vi "PhotronPDCMessageLoop.vi"(8 "Error In":errorcluster, 11 "CommunicationRefs":T1) -> (0 "Error Out":errorcluster)   [LabVIEW 2015]
uses:
  TypeDefs/CommunicationRefs.ctl
  TypeDefs/MessageCluster.ctl
  TypeDefs/PDCSettings.ctl
  TypeDefs/PDCRecordStatus.ctl
  TypeDefs/PDCAllStates.ctl
  TypeDefs/PDCDisplay.ctl
  TypeDefs/PDCSaveSettings.ctl
  TypeDefs/PDCLists.ctl
  TypeDefs/PDCSetup.ctl
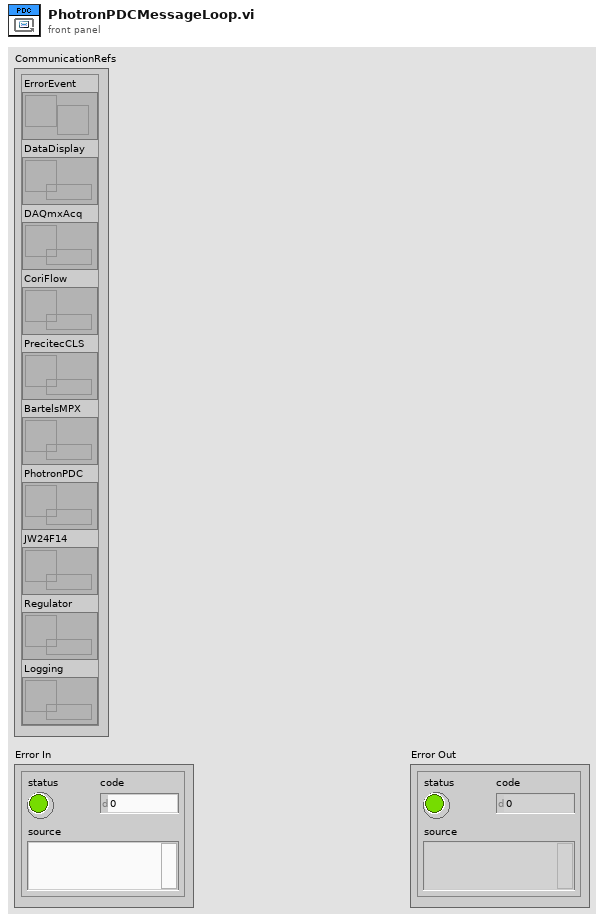
[diagram p1: front panel]
types:
  T1 = typedef "CommunicationRefs.ctl" = cluster{"ErrorEvent":refnum<user-event>, "DataDisplay":refnum<queue>, "DAQmxAcq":refnum<queue>, "CoriFlow":refnum<queue>, "PrecitecCLS":refnum<queue>, "BartelsMPX":refnum<queue>, "PhotronPDC":refnum<queue>, "JW24F14":refnum<queue>, "Regulator":refnum<queue>, "Logging":refnum<queue>}
  T2 = typedef "PDCRecordStatus.ctl" = enum16{"Live", "Endless", "Recording"}
  T3 = typedef "PDCSaveSettings.ctl" = cluster{"Save Folder":path, "File Name":string, "Data Type":enum16{"BMP", "AVI", "MRAW"}}
  T4 = cluster{"PDC Save Settings":T3, "SaveStatus":refnum<vi>}
  T5 = typedef "PDCAllStates.ctl" = cluster{"DeviceNo":u32, "ChildNo":u32, "ColorType":enum16{"MONO", "COLOR"}, "BitDepth":i8, "Resolution":cluster{"Width":u32, "Height":u32}, "RecordRate":u32, "ShutterSpeed":u32, "TriggerMode":u32, "Display":T6, "PDCRecordStatus":T2, "PlayFrames":bool, "Start Frame":i32, "Current Frame":i32, "End Frame":i32, "RefImage8bit":u8[], "RefImage16bit":u16[], "Auto Trigger":bool, "PDCSettings":T7}
  T6 = typedef "PDCDisplay.ctl" = enum16{"Live", "Memory", "LiveStop"}
  T7 = typedef "PDCSettings.ctl" = cluster{"Interface":enum16{"Gigabit-Ethernet", "IEEE1394a", "Photron Optical", "PCI/PCI Express"}, "AutoSearch":bool, "IP - AutoSearch":u32[], "IP - Direct":u32[], "Simulate":bool}
  T8 = typedef "PDCLists.ctl" = cluster{"ResolutionList":string[], "RecordRateList":string[], "ShutterSpeedList":string[], "TriggerModeList":string[]}
  T9 = typedef "PDCSetup.ctl" = cluster{"Color Type":enum16{"MONO", "COLOR"}, "Bit Depth":i8, "Resolution":u16, "Record Rate":u16, "Shutter Speed":u16, "Trigger Mode":u16, "Display":T6, "Auto Trigger":bool}
  T10 = cluster{"Start":i32, "End":i32, "Trigger":i32, "TwoStageLowToHigh":i32, "TwoStageHighToLow":i32, "TwoStageTiming":u32, "Event":i32[], "EventCount":u32, "RecordedFrames":u32}
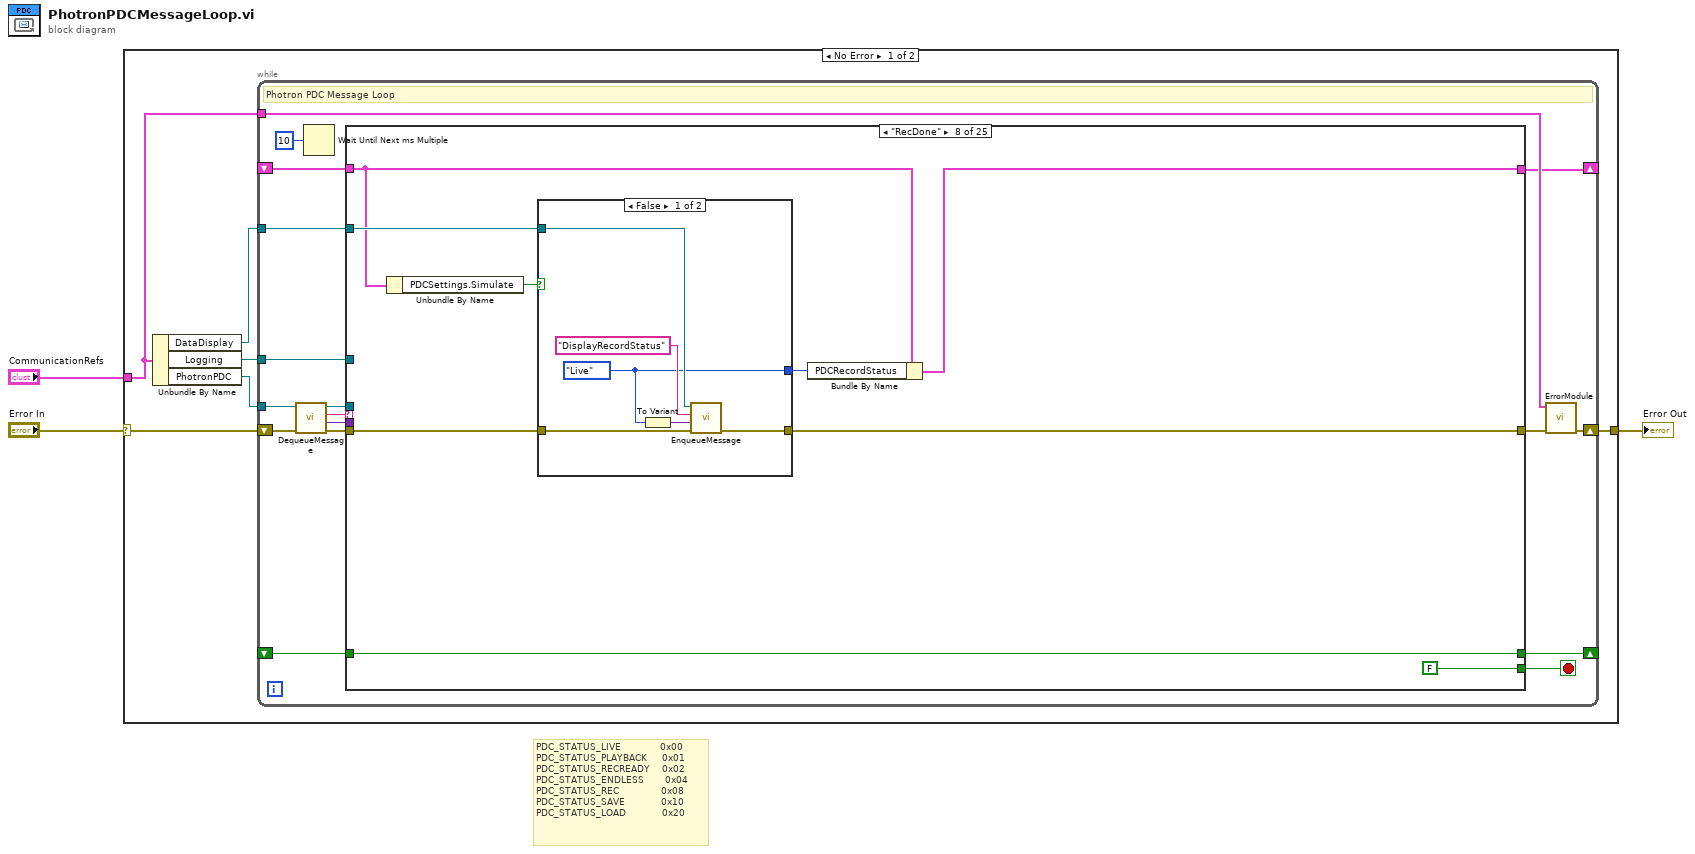
[diagram p0: block diagram]
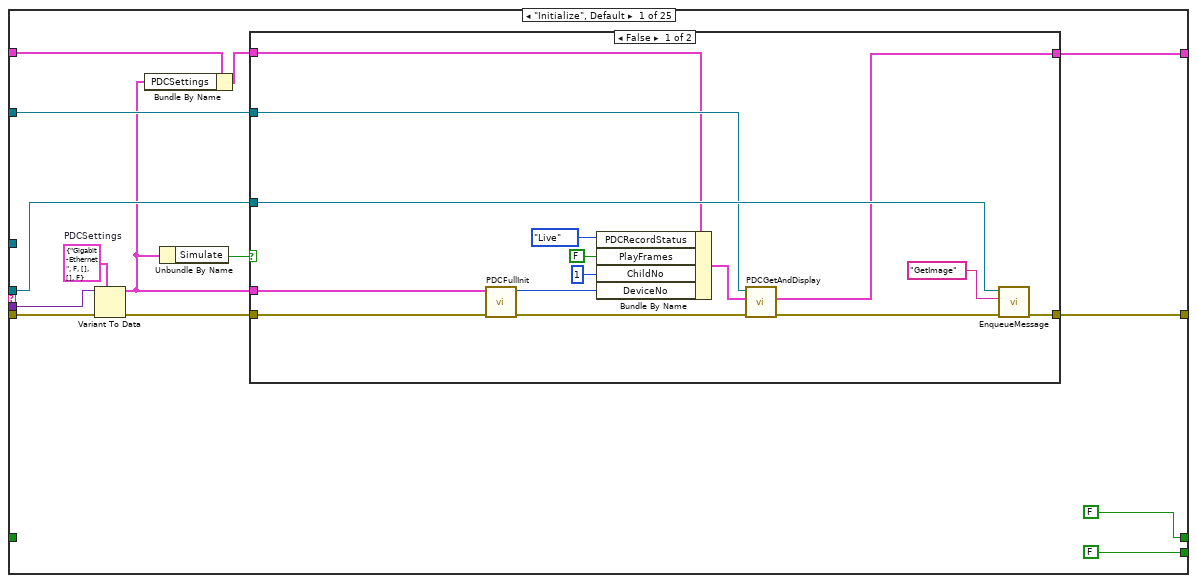
[diagram p2: hidden frame]
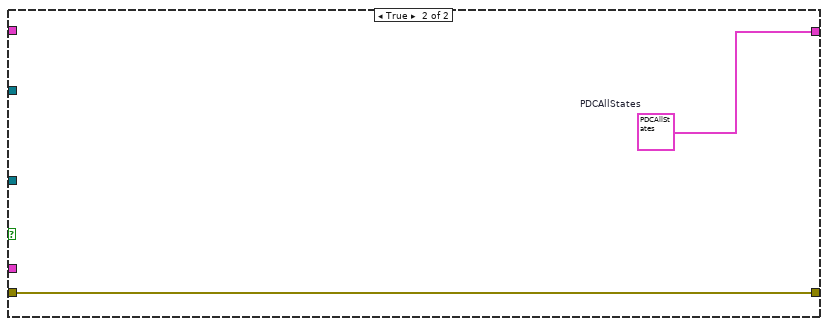
[diagram p3: hidden frame]
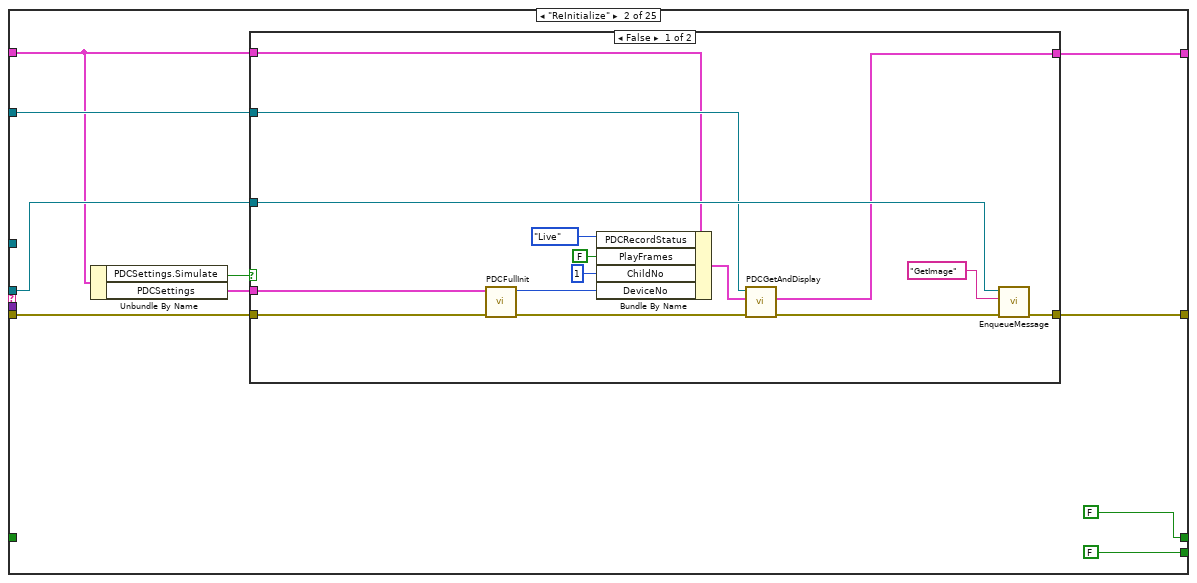
[diagram p4: hidden frame]
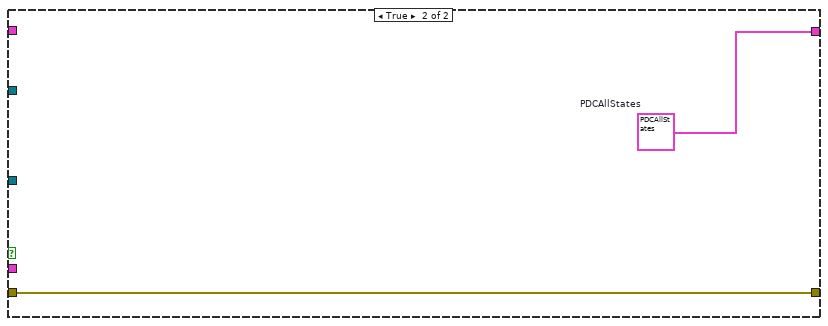
[diagram p5: hidden frame]
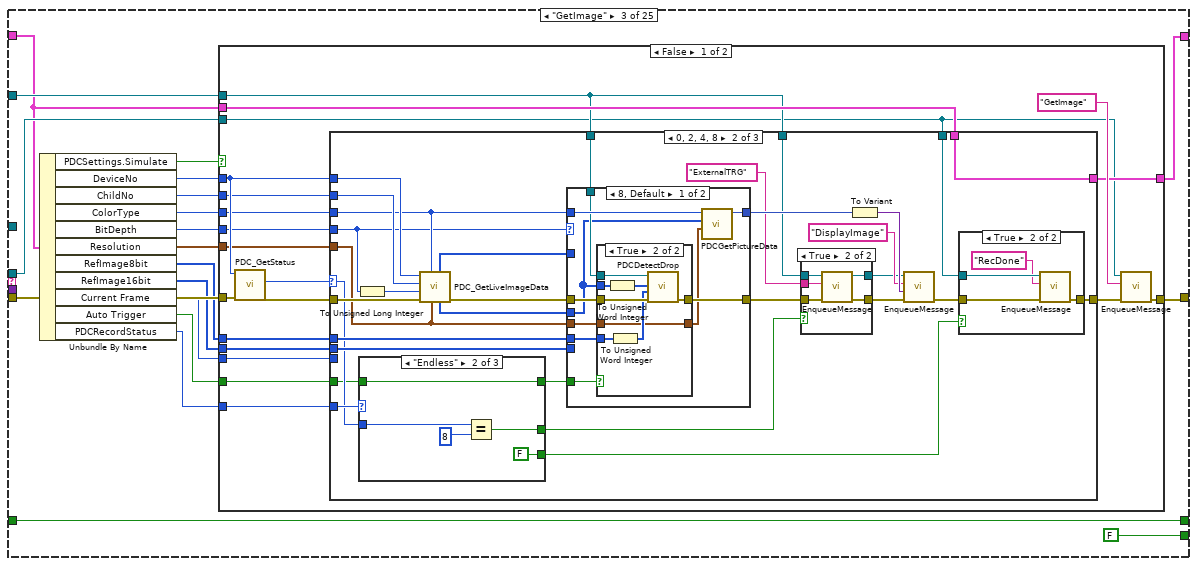
[diagram p6: hidden frame]
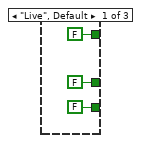
[diagram p9: hidden frame]
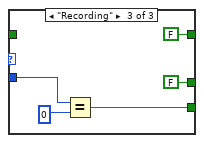
[diagram p10: hidden frame]
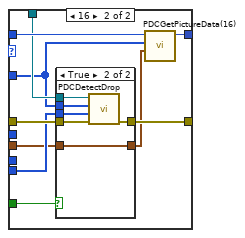
[diagram p13: hidden frame]
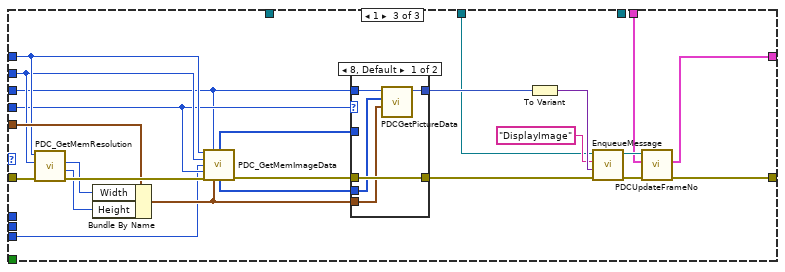
[diagram p15: hidden frame]
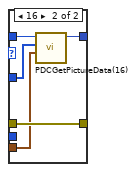
[diagram p16: hidden frame]
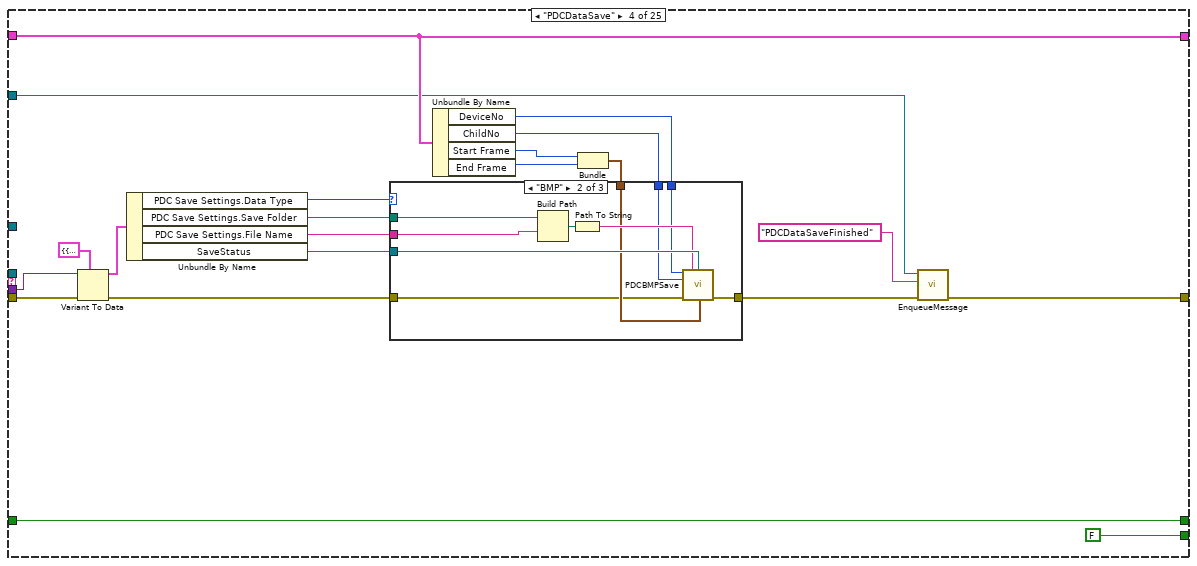
[diagram p18: hidden frame]
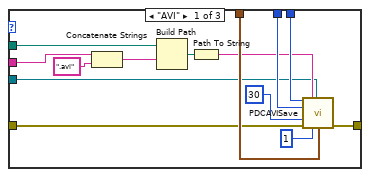
[diagram p19: hidden frame]
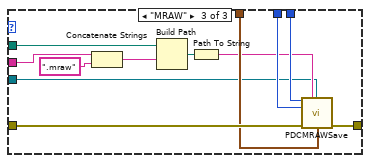
[diagram p20: hidden frame]
diagram:
  # "PDC_STATUS_LIVE\t\t\t\t\t\t       0x00\nPDC_STATUS_PLAYBACK\t\t\t\t\t0x01\nPDC_STATUS_RECREADY\t\t\t\t0x02\nPDC_STATUS_ENDLESS\t\t\t\t\t  0x04\nPDC_STATUS_REC\t\t\t\t\t\t        0x08\nPDC_STATUS_SAVE\t\t\t\t\t       0x10\nPDC_STATUS_LOAD\t\t\t\t\t\t      0x20"
  n1 = case shown="No Error" "Error In" {
    selector: "Error In" -> [w8 w753]
    tunnel: [w7 w753] -> w2
    tunnel: "CommunicationRefs" -> [w6 _]
    frame No Error {
      n2 = Unbundle By Name(w6) -> ("DataDisplay"=w5:refnum<queue>, "Logging"=w4:refnum<queue>, "PhotronPDC"=w9:refnum<queue>)
      n3 = while {
        tunnel: w9 -> [w26]
        tunnel: w6 -> [w18]
        shift-right: [w20] -> w7
        shift-left: w8 -> [w25]
        tunnel: w5 -> [w16]
        tunnel: w4 -> [w15]
        shift-right: [w14] -> _
        shift-left: _ -> [w13]
        shift-right: [w12] -> _
        shift-left: _ -> [w11]
        stop <- w17 stop-if-true
        # "Photron PDC Message Loop"
        n4 = call "DequeueMessage.vi"("error in (no error)"=w25, "MessageQueue"=w26) -> ("error out"=w21:errorcluster, "MessageData"=w22:variant, "Message"=w23:string, "dupMessageQueue"=w24:refnum<queue>)  [unwired: 6 in]
        n5 = Wait Until Next ms Multiple(millisecond multiple=u32 10) -> ()  [unwired: 1 out]
        n6 = case shown="\"RecDone\"" w23 {
          tunnel: w24 -> [w33 w63 w93 _ w313 w357 _ _ _ _ _ _ _ _ _ _ _ _ _ _ _ _ _ _ w742]
          tunnel: w22 -> [w30 _ _ w267 w321 _ _ _ w428 w437 w448 w457 w466 w480 w525 w577 w602 w627 w654 w679 w704 _ _ _ _]
          tunnel: w21 -> [w37 w58 w101 w268 w323 w364 w395 w415 w436 w445 w454 w463 w472 w482 w527 w579 w604 w629 w656 w681 w706 w721 w728 w733 w741]
          tunnel: [w38 w65 w95 w259 w324 w358 w396 w416 w431 w440 w451 w460 w469 w484 w529 w581 w606 w631 w658 w683 w708 w721 w728 w732 w747] -> w19
          tunnel: [FALSE FALSE FALSE FALSE FALSE FALSE FALSE FALSE FALSE FALSE FALSE FALSE FALSE FALSE FALSE FALSE FALSE FALSE FALSE FALSE FALSE FALSE FALSE TRUE FALSE] -> w17
          tunnel: w16 -> [w34 w64 w94 w257 w317 _ w393 w414 _ _ _ _ _ w475 w519 w572 w597 w623 w649 w674 w699 _ _ _ _]
          tunnel: w15 -> [_ _ _ _ _ _ _ _ _ _ _ _ _ _ _ _ _ _ _ _ _ _ _ _ _]
          tunnel: [FALSE FALSE w91 w275 w327 w354 w399 w419 w430 w439 w450 w459 w468 w486 w531 w583 w608 w633 w660 w685 w710 TRUE FALSE FALSE w743] -> w14
          tunnel: w13 -> [_ _ w91 w275 w327 w354 w399 w419 w430 w439 w450 w459 w468 w486 w531 w583 w608 w633 w660 w685 w710 _ _ _ w743]
          tunnel: [w31 w61 w92 w274 w315 w355 w391 w412 w432 w441 w452 w461 w470 w477 w521 w574 w599 w625 w651 w676 w701 w722 w725 w731 w746] -> w12
          tunnel: w11 -> [w29 w60 w87 w274 w316 w356 w392 w413 w434 w443 w453 w462 w471 w474 w518 w570 w595 w620 w647 w672 w697 w722 w725 w731 w746]
          frame "Initialize", Default {
            w35 = T7 {"Interface"=enum."Gigabit-Ethernet", "AutoSearch"=FALSE, "IP - AutoSearch"=[], "IP - Direct"=[], "Simulate"=FALSE}  # PDCSettings
            n7 = Variant To Data(error in=w37, type=w35, Variant=w30) -> (data=w28:T7, error out=w36:errorcluster)
            n8 = Bundle By Name(cluster=w29, "PDCSettings"=w28) -> (w27:T5)
            n9 = Unbundle By Name(w28) -> ("Simulate"=w32:bool)
            n10 = case shown="False" w32 {
              tunnel: [w52 w57] -> w38
              tunnel: w36 -> [w54 w57]
              tunnel: w34 -> [w48 _]
              tunnel: w33 -> [w53 _]
              tunnel: [w50 w56] -> w31
              tunnel: w28 -> [w47 _]
              tunnel: w27 -> [w43 _]
              frame False {
                n11 = call "PDCFullInit.vi"("error in (no error)"=w54, "PDCSettings"=w47) -> ("error out"=w49:errorcluster, "DeviceNo"=w46:u32)  [unwired: 8 in]
                n12 = Bundle By Name(cluster=w43, "PDCRecordStatus"=PDCRecordStatus."Live", "PlayFrames"=FALSE, "ChildNo"=u32 1, "DeviceNo"=w46) -> (w44:T5)
                n13 = call "PDCGetAndDisplay.vi"("error in (no error)"=w49, "PDCAllStates in"=w44, "DataDisplayQueue"=w48) -> ("error out"=w55:errorcluster, "PDCAllStates out"=w50:T5)  [unwired: 7 in]
                n14 = call "EnqueueMessage.vi"("error in (no error)"=w55, "Message"="GetImage", "MessageQueue"=w53) -> ("error out"=w52:errorcluster)  [unwired: 7 in, 1 out]
              }
              frame True {
                w56 = T5 {"DeviceNo"=0, "ChildNo"=1, "ColorType"=enum."MONO", "BitDepth"=0, "Resolution"={"Width"=0, "Height"=0}, "RecordRate"=0, "ShutterSpeed"=0, "TriggerMode"=0, "Display"=enum."LiveStop", "PDCRecordStatus"=enum."Live", "PlayFrames"=FALSE, "Start Frame"=0, "Current Frame"=0, "End Frame"=0, "RefImage8bit"=[], "RefImage16bit"=[], "Auto Trigger"=FALSE, "PDCSettings"={"Interface"=enum."Gigabit-Ethernet", "AutoSearch"=FALSE, "IP - AutoSearch"=[], "IP - Direct"=[], "Simulate"=FALSE}}  # PDCAllStates
              }
            }
          }
          frame "ReInitialize" {
            n15 = Unbundle By Name(w60) -> ("PDCSettings.Simulate"=w62:bool, "PDCSettings"=w59:T7)
            n16 = case shown="False" w62 {
              tunnel: [w79 w84] -> w65
              tunnel: w58 -> [w81 w84]
              tunnel: w64 -> [w75 _]
              tunnel: w63 -> [w80 _]
              tunnel: [w77 w83] -> w61
              tunnel: w59 -> [w74 _]
              tunnel: w60 -> [w70 _]
              frame False {
                n17 = call "PDCFullInit.vi"("error in (no error)"=w81, "PDCSettings"=w74) -> ("error out"=w76:errorcluster, "DeviceNo"=w73:u32)  [unwired: 8 in]
                n18 = Bundle By Name(cluster=w70, "PDCRecordStatus"=PDCRecordStatus."Live", "PlayFrames"=FALSE, "ChildNo"=u32 1, "DeviceNo"=w73) -> (w71:T5)
                n19 = call "PDCGetAndDisplay.vi"("error in (no error)"=w76, "PDCAllStates in"=w71, "DataDisplayQueue"=w75) -> ("error out"=w82:errorcluster, "PDCAllStates out"=w77:T5)  [unwired: 7 in]
                n20 = call "EnqueueMessage.vi"("error in (no error)"=w82, "Message"="GetImage", "MessageQueue"=w80) -> ("error out"=w79:errorcluster)  [unwired: 7 in, 1 out]
              }
              frame True {
                w83 = T5 {"DeviceNo"=0, "ChildNo"=1, "ColorType"=enum."MONO", "BitDepth"=0, "Resolution"={"Width"=0, "Height"=0}, "RecordRate"=0, "ShutterSpeed"=0, "TriggerMode"=0, "Display"=enum."LiveStop", "PDCRecordStatus"=enum."Live", "PlayFrames"=FALSE, "Start Frame"=0, "Current Frame"=0, "End Frame"=0, "RefImage8bit"=[], "RefImage16bit"=[], "Auto Trigger"=FALSE, "PDCSettings"={"Interface"=enum."Gigabit-Ethernet", "AutoSearch"=FALSE, "IP - AutoSearch"=[], "IP - Direct"=[], "Simulate"=FALSE}}  # PDCAllStates
              }
            }
          }
          frame "GetImage" {
            n21 = Unbundle By Name(w87) -> ("PDCSettings.Simulate"=w102:bool, "DeviceNo"=w100:u32, "ChildNo"=w99:u32, "ColorType"=w98:enum16{"MONO", "COLOR"}, "BitDepth"=w97:i8, "Resolution"=w96:cluster{"Width":u32, "Height":u32}, "RefImage8bit"=w88:u8[], "RefImage16bit"=w89:u16[], "Current Frame"=w90:i32, "Auto Trigger"=w85:bool, "PDCRecordStatus"=w86:T2)
            n22 = case shown="False" w102 {
              tunnel: w101 -> [w123 w255]
              tunnel: w100 -> [w122 _]
              tunnel: w99 -> [w121 _]
              tunnel: w98 -> [w118 _]
              tunnel: w97 -> [w119 _]
              tunnel: w96 -> [w116 _]
              tunnel: [w115 w255] -> w95
              tunnel: w94 -> [w107 _]
              tunnel: w93 -> [w104 _]
              tunnel: w87 -> [w112 w254]
              tunnel: [w111 w254] -> w92
              tunnel: w90 -> [w110 _]
              tunnel: w89 -> [w109 _]
              tunnel: w88 -> [w108 _]
              tunnel: w86 -> [w106 _]
              tunnel: w85 -> [w105 _]
              frame False {
                n23 = call "PDC_GetStatus.vi"("error in (no error)"=w123, "DeviceNo"=w122) -> ("error out"=w120:errorcluster, "Status"=w117:u32)  [unwired: 6 in, 2 out]
                n24 = case shown="0, 2, 4, 8" w117 {
                  selector: w117 -> [_ w133 _]
                  tunnel: w122 -> [_ w156 w238]
                  tunnel: w121 -> [_ w155 w237]
                  tunnel: w120 -> [w125 w154 w242]
                  tunnel: w119 -> [_ w147 w233]
                  tunnel: w118 -> [_ w148 w232]
                  tunnel: w116 -> [_ w151 w241]
                  tunnel: [w125 w128 w224] -> w113
                  tunnel: w107 -> [_ w142 w226]
                  tunnel: w112 -> [w124 w138 w222]
                  tunnel: [w124 w138 w221] -> w111
                  tunnel: w110 -> [_ _ w220]
                  tunnel: w109 -> [_ w136 _]
                  tunnel: w108 -> [_ w137 _]
                  tunnel: w107 -> [_ w135 _]
                  tunnel: w105 -> [_ w132 _]
                  tunnel: w106 -> [_ w134 _]
                  tunnel: w104 -> [_ w126 _]
                  frame Default {
                  }
                  frame 0, 2, 4, 8 {
                    n25 = To Unsigned Long Integer(number=w147) -> (unsigned 32bit integer=w153:u32)
                    n26 = case shown="\"Endless\"" w134 {
                      tunnel: w133 -> [_ w167 w171]
                      tunnel: w132 -> [_ w169 _]
                      tunnel: [FALSE ("Auto Trigger") w169 FALSE ("Auto Trigger")] -> w131
                      tunnel: [FALSE w166 FALSE] -> w130
                      tunnel: [FALSE FALSE w170] -> w127
                      frame "Live", Default {
                      }
                      frame "Endless" {
                        n27 = Equal?(x=w167, y=u32 8) -> (x = y?=w166:bool)
                      }
                      frame "Recording" {
                        n28 = Equal?(x=w171, y=u32 0) -> (x = y?=w170:bool)
                      }
                    }
                    n29 = call "PDC_GetLiveImageData.vi"("Resolution"=w151, "ColorType"=w148, "error in (no error)"=w154, "BitDepth"=w153, "ChildNo"=w155, "DeviceNo"=w156) -> ("error out"=w152:errorcluster, "Data(8Bit)"=w150:u8[], "Data(16Bit)"=w149:u16[])  [unwired: 1 in, 2 out]
                    n30 = case shown="8, Default" w147 {
                      tunnel: w148 -> [w191 w211]
                      tunnel: w151 -> [w183 w203]
                      tunnel: w150 -> [w185 _]
                      tunnel: w152 -> [w189 w209]
                      tunnel: [w188 w208] -> w140
                      tunnel: w149 -> [_ w205]
                      tunnel: [w190 w210] -> w144
                      tunnel: w137 -> [w186 _]
                      tunnel: w136 -> [_ w206]
                      tunnel: w135 -> [w187 w207]
                      tunnel: w131 -> [w184 w204]
                      frame 8, Default {
                        n31 = case shown="True" w184 {
                          tunnel: w189 -> [w192 w201]
                          tunnel: [w192 w200] -> w188
                          tunnel: w187 -> [_ w199]
                          tunnel: w186 -> [_ w198]
                          tunnel: w185 -> [_ w196]
                          tunnel: w183 -> [w193 w194]
                          tunnel: [w193 w194] -> w182
                          frame False {
                          }
                          frame True {
                            n32 = To Unsigned Word Integer(number=w196) -> (unsigned 16bit integer=w195:u16[])
                            n33 = To Unsigned Word Integer(number=w198) -> (unsigned 16bit integer=w197:u16[])
                            n34 = call "PDCDetectDrop.vi"("Error In"=w201, "RefImage"=w197, "CurrentImage"=w195, "DataDisplay"=w199) -> ("Error Out"=w200:errorcluster)  [unwired: 7 in]
                          }
                        }
                        n35 = call "PDCGetPictureData.vi"("Resolution"=w182, "Data(8Bit)"=w185, "ColorType"=w191) -> ("new picture"=w190:picture)  [unwired: 4 in]
                      }
                      frame 16 {
                        n36 = case shown="True" w204 {
                          tunnel: w209 -> [w212 w219]
                          tunnel: [w212 w218] -> w208
                          tunnel: w207 -> [_ w217]
                          tunnel: w206 -> [_ w216]
                          tunnel: w205 -> [_ w215]
                          tunnel: [w213 w214] -> w202
                          tunnel: w203 -> [w213 w214]
                          frame False {
                          }
                          frame True {
                            n37 = call "PDCDetectDrop.vi"("Error In"=w219, "RefImage"=w216, "CurrentImage"=w215, "DataDisplay"=w217) -> ("Error Out"=w218:errorcluster)  [unwired: 7 in]
                          }
                        }
                        n38 = call "PDCGetPictureData(16).vi"("Resolution"=w202, "Data(16Bit)"=w205, "ColorType"=w211) -> ("new picture"=w210:picture)  [unwired: 4 in]
                      }
                    }
                    n39 = case shown="True" w130 {
                      tunnel: [w176 w181] -> w143
                      tunnel: w142 -> [w175 w178]
                      tunnel: [w175 w177] -> w141
                      tunnel: w140 -> [w176 w180]
                      tunnel: "ExternalTRG" ("Message") -> [_ w179]
                      frame False {
                      }
                      frame True {
                        n40 = call "EnqueueMessage.vi"("error in (no error)"=w180, "Message"=w179, "MessageQueue"=w178) -> ("error out"=w181:errorcluster, "dupMessageQueue"=w177:refnum<queue>)  [unwired: 7 in]
                      }
                    }
                    n41 = To Variant(anything=w144) -> (Variant=w146:variant)
                    n42 = call "EnqueueMessage.vi"("error in (no error)"=w143, "MessageData"=w146, "Message"="DisplayImage", "MessageQueue"=w141) -> ("error out"=w129:errorcluster)  [unwired: 6 in, 1 out]
                    n43 = case shown="True" w127 {
                      tunnel: w126 -> [_ w161]
                      tunnel: w129 -> [w157 w160]
                      tunnel: [w157 w159] -> w128
                      frame False {
                      }
                      frame True {
                        n44 = call "EnqueueMessage.vi"("error in (no error)"=w160, "Message"="RecDone", "MessageQueue"=w161) -> ("error out"=w159:errorcluster)  [unwired: 7 in, 1 out]
                      }
                    }
                  }
                  frame 1 {
                    n45 = call "PDC_GetMemResolution.vi"("error in (no error)"=w242, "ChildNo"=w237, "DeviceNo"=w238) -> ("error out"=w243:errorcluster, "Height"=w240:u32, "Width"=w239:u32)  [unwired: 4 in, 2 out]
                    n46 = Bundle By Name(cluster=w241, "Width"=w239, "Height"=w240) -> (w235:cluster{"Width":u32, "Height":u32})
                    n47 = call "PDC_GetMemImageData.vi"("DeviceNo"=w238, "ColorType"=w232, "ChildNo"=w237, "FrameNo"=w220, "BitDepth"=w233, "error in (no error)"=w243, "Resolution"=w235) -> ("Data(16Bit)"=w231:u16[], "Data(8Bit)"=w234:u8[], "error out"=w236:errorcluster)  [unwired: 4 in, 2 out]
                    n48 = case shown="8, Default" w233 {
                      tunnel: w232 -> [w247 w252]
                      tunnel: w235 -> [w246 w251]
                      tunnel: w234 -> [w245 _]
                      tunnel: w236 -> [w248 w253]
                      tunnel: [w248 w253] -> w230
                      tunnel: w231 -> [_ w250]
                      tunnel: [w244 w249] -> w229
                      frame 8, Default {
                        n49 = call "PDCGetPictureData.vi"("Resolution"=w246, "Data(8Bit)"=w245, "ColorType"=w247) -> ("new picture"=w244:picture)  [unwired: 4 in]
                      }
                      frame 16 {
                        n50 = call "PDCGetPictureData(16).vi"("Resolution"=w251, "Data(16Bit)"=w250, "ColorType"=w252) -> ("new picture"=w249:picture)  [unwired: 4 in]
                      }
                    }
                    n51 = To Variant(anything=w229) -> (Variant=w228:variant)
                    n52 = call "EnqueueMessage.vi"("error in (no error)"=w230, "MessageData"=w228, "Message"="DisplayImage", "MessageQueue"=w226) -> ("error out"=w225:errorcluster, "dupMessageQueue"=w223:refnum<queue>)  [unwired: 6 in]
                    n53 = call "PDCUpdateFrameNo.vi"("Error In"=w225, "PDCAllStates in"=w222, "DataDisplayQueue"=w223) -> ("Error Out"=w224:errorcluster, "PDCAllStates out"=w221:T5)  [unwired: 7 in]
                  }
                }
                n54 = call "EnqueueMessage.vi"("error in (no error)"=w113, "Message"="GetImage", "MessageQueue"=w104) -> ("error out"=w115:errorcluster)  [unwired: 7 in, 1 out]
              }
              frame True {
              }
            }
          }
          frame "PDCDataSave" {
            n55 = Variant To Data(error in=w268, type=T4 {"PDC Save Settings"={"Save Folder"=path "", "File Name"="", "Data Type"=enum."AVI"}, "SaveStatus"=refnum} ("cluster"), Variant=w267) -> (data=w265:T4, error out=w264:errorcluster)
            n56 = Unbundle By Name(w265) -> ("PDC Save Settings.Data Type"=w260:enum16{"BMP", "AVI", "MRAW"}, "PDC Save Settings.Save Folder"=w262:path, "PDC Save Settings.File Name"=w261:string, "SaveStatus"=w263:refnum<vi>)
            n57 = Unbundle By Name(w274) -> ("DeviceNo"=w273:u32, "ChildNo"=w272:u32, "Start Frame"=w271:i32, "End Frame"=w270:i32)
            n58 = Bundle("Start Frame"=w271, "End Frame"=w270) -> (w269:cluster{"Start Frame":i32, "End Frame":i32})  [unwired: 1 in]
            n59 = case shown="\"BMP\"" w260 {
              tunnel: [w290 w294 w307] -> w258
              tunnel: w273 -> [w289 w296 w303]
              tunnel: w272 -> [w288 w295 w304]
              tunnel: w269 -> [w287 w293 w305]
              tunnel: w264 -> [w282 w292 w306]
              tunnel: w263 -> [w281 w298 w301]
              tunnel: w262 -> [w280 w299 w311]
              tunnel: w261 -> [w279 w291 w310]
              frame "AVI" {
                n60 = Concatenate Strings(w279, ".avi" ("string")) -> (w278:string)
                n61 = Build Path(base path=w280, name or relative path=w278) -> (appended path=w284:path)
                n62 = Path To String(path=w284) -> (string=w283:string)
                n63 = call "PDCAVISave.vi"("DeviceNo"=w289, "FileName"=w283, "Slide Refnum"=w281, "ChildNo"=w288, "Rate"=30, "error in (no error)"=w282, "ShowCompreddDlg"=u32 1, "File_Frame"=w287) -> ("error out"=w290:errorcluster)  [unwired: 7 in]
              }
              frame "BMP" {
                n64 = Build Path(base path=w299, name or relative path=w291) -> (appended path=w300:path)
                n65 = Path To String(path=w300) -> (string=w297:string)
                n66 = call "PDCBMPSave.vi"("DeviceNo"=w296, "FileName"=w297, "Slide Refnum"=w298, "ChildNo"=w295, "error in (no error)"=w292, "File_Frame"=w293) -> ("error out"=w294:errorcluster)  [unwired: 9 in]
              }
              frame "MRAW" {
                n67 = Concatenate Strings(w310, ".mraw" ("string")) -> (w309:string)
                n68 = Build Path(base path=w311, name or relative path=w309) -> (appended path=w312:path)
                n69 = Path To String(path=w312) -> (string=w302:string)
                n70 = call "PDCMRAWSave.vi"("DeviceNo"=w303, "FileName"=w302, "Slide Refnum"=w301, "ChildNo"=w304, "error in (no error)"=w306, "File_Frame"=w305) -> ("error out"=w307:errorcluster)  [unwired: 9 in]
              }
            }
            n71 = call "EnqueueMessage.vi"("error in (no error)"=w258, "Message"="PDCDataSaveFinished", "MessageQueue"=w257) -> ("error out"=w259:errorcluster)  [unwired: 7 in, 1 out]
          }
          frame "Record" {
            n72 = Unbundle By Name(w316) -> ("PDCSettings.Simulate"=w325:bool, "DeviceNo"=w318:u32)
            n73 = Variant To Data(error in=w323, type=PDCRecordStatus."Live" ("PDCRecordState"), Variant=w321) -> (data=w319:T2, error out=w322:errorcluster)
            n74 = case shown="False" w325 {
              tunnel: w322 -> [w335 w353]
              tunnel: [w333 w353] -> w324
              tunnel: w319 -> [w337 _]
              tunnel: w318 -> [w336 _]
              tunnel: w317 -> [w332 _]
              tunnel: [w329 PDCRecordStatus."Live" ("PDCRecordState")] -> w314
              tunnel: w313 -> [w328 _]
              frame False {
                n75 = case shown="\"Live\", Default" w337 {
                  tunnel: w336 -> [w339 w347 _]
                  tunnel: w335 -> [w340 w349 w351]
                  tunnel: [w344 w348 w351] -> w334
                  tunnel: [PDCRecordStatus."Endless" ("PDCRecordState") PDCRecordStatus."Recording" ("PDCRecordState") PDCRecordStatus."Recording" ("PDCRecordState")] -> w329
                  tunnel: w328 -> [w343 _ _]
                  frame "Live", Default {
                    n76 = call "PDC_SetEndless.vi"("error in (no error)"=w340, "DeviceNo"=w339) -> ("error out"=w338:errorcluster)  [unwired: 7 in, 2 out]
                    n77 = call "EnqueueMessage.vi"("Priority Message? (F)"=TRUE, "error in (no error)"=w338, "Message"="SetRefImage", "MessageQueue"=w343) -> ("error out"=w344:errorcluster)  [unwired: 6 in, 1 out]
                  }
                  frame "Endless" {
                    n78 = call "PDC_TriggerIn.vi"("error in (no error)"=w349, "DeviceNo"=w347) -> ("error out"=w348:errorcluster)  [unwired: 7 in, 2 out]
                  }
                  frame "Recording" {
                  }
                }
                n79 = To Variant(anything=w329) -> (Variant=w330:variant)
                n80 = call "EnqueueMessage.vi"("error in (no error)"=w334, "MessageData"=w330, "Message"="DisplayRecordStatus", "MessageQueue"=w332) -> ("error out"=w333:errorcluster)  [unwired: 6 in, 1 out]
              }
              frame True {
              }
            }
            n81 = Bundle By Name(cluster=w316, "PDCRecordStatus"=w314) -> (w315:T5)
          }
          frame "SetRefImage" {
            n82 = Unbundle By Name(w356) -> ("PDCSettings.Simulate"=w365:bool, "DeviceNo"=w363:u32, "ChildNo"=w362:u32, "ColorType"=w361:enum16{"MONO", "COLOR"}, "BitDepth"=w360:i8, "Resolution"=w359:cluster{"Width":u32, "Height":u32})
            n83 = case shown="False" w365 {
              tunnel: w364 -> [w370 w389]
              tunnel: w363 -> [w379 _]
              tunnel: w362 -> [w378 _]
              tunnel: w361 -> [w376 _]
              tunnel: w360 -> [w377 _]
              tunnel: w359 -> [w375 _]
              tunnel: [w369 w389] -> w358
              tunnel: w357 -> [_ _]
              tunnel: w356 -> [w368 w388]
              tunnel: [w367 w388] -> w355
              frame False {
                n84 = To Unsigned Long Integer(number=w377) -> (unsigned 32bit integer=w374:u32)
                n85 = call "PDC_GetLiveImageData.vi"("Resolution"=w375, "ColorType"=w376, "error in (no error)"=w370, "BitDepth"=w374, "ChildNo"=w378, "DeviceNo"=w379) -> ("error out"=w373:errorcluster, "Data(8Bit)"=w372:u8[], "Data(16Bit)"=w371:u16[])  [unwired: 1 in, 2 out]
                n86 = case shown="8, Default" w377 {
                  tunnel: w376 -> [_ _]
                  tunnel: w372 -> [w381 _]
                  tunnel: w373 -> [w383 w387]
                  tunnel: [w383 w387] -> w369
                  tunnel: w371 -> [_ w384]
                  tunnel: w368 -> [w382 w386]
                  tunnel: [w380 w385] -> w367
                  frame 8, Default {
                    n87 = Bundle By Name(cluster=w382, "RefImage8bit"=w381) -> (w380:T5)
                  }
                  frame 16 {
                    n88 = Bundle By Name(cluster=w386, "RefImage16bit"=w384) -> (w385:T5)
                  }
                }
              }
              frame True {
              }
            }
          }
          frame "RecStop" {
            n89 = Unbundle By Name(w392) -> ("PDCSettings.Simulate"=w397:bool, "DeviceNo"=w394:u32)
            n90 = case shown="False" w397 {
              tunnel: w395 -> [w402 w410]
              tunnel: [w408 w410] -> w396
              tunnel: w394 -> [w401 _]
              tunnel: w393 -> [w407 _]
              tunnel: [w404 PDCRecordStatus."Live" ("PDCRecordState")] -> w390
              frame False {
                w400 = u32 0  # STATUS LIVE
                w404 = PDCRecordStatus."Live" ("PDCRecordState")
                n91 = call "PDC_SetStatus.vi"("error in (no error)"=w402, "Mode"=w400, "DeviceNo"=w401) -> ("error out"=w403:errorcluster)  [unwired: 6 in, 2 out]
                n92 = To Variant(anything=w404) -> (Variant=w405:variant)
                n93 = call "EnqueueMessage.vi"("error in (no error)"=w403, "MessageData"=w405, "Message"="DisplayRecordStatus", "MessageQueue"=w407) -> ("error out"=w408:errorcluster)  [unwired: 6 in, 1 out]
              }
              frame True {
              }
            }
            n94 = Bundle By Name(cluster=w392, "PDCRecordStatus"=w390) -> (w391:T5)
          }
          frame "RecDone" {
            n95 = Unbundle By Name(w413) -> ("PDCSettings.Simulate"=w417:bool)
            n96 = case shown="False" w417 {
              tunnel: w415 -> [w420 w427]
              tunnel: [w425 w427] -> w416
              tunnel: w414 -> [w424 _]
              tunnel: [w421 PDCRecordStatus."Live" ("PDCRecordState")] -> w411
              frame False {
                w421 = PDCRecordStatus."Live" ("PDCRecordState")
                n97 = To Variant(anything=w421) -> (Variant=w422:variant)
                n98 = call "EnqueueMessage.vi"("error in (no error)"=w420, "MessageData"=w422, "Message"="DisplayRecordStatus", "MessageQueue"=w424) -> ("error out"=w425:errorcluster)  [unwired: 6 in, 1 out]
              }
              frame True {
              }
            }
            n99 = Bundle By Name(cluster=w413, "PDCRecordStatus"=w411) -> (w412:T5)
          }
          frame "TogglePlayFrames" {
            n100 = Variant To Data(error in=w436, type=FALSE, Variant=w428) -> (data=w433:bool, error out=w431:errorcluster)
            n101 = Bundle By Name(cluster=w434, "PlayFrames"=w433) -> (w432:T5)
          }
          frame "ToggleAutoTrigger" {
            n102 = Variant To Data(error in=w445, type=FALSE, Variant=w437) -> (data=w442:bool, error out=w440:errorcluster)
            n103 = Bundle By Name(cluster=w443, "Auto Trigger"=w442) -> (w441:T5)
          }
          frame "UpdateCurrentFrame" {
            n104 = Variant To Data(error in=w454, type=0 ("Current Frame"), Variant=w448) -> (data=w446:i32, error out=w451:errorcluster)
            n105 = Bundle By Name(cluster=w453, "Current Frame"=w446) -> (w452:T5)
          }
          frame "UpdateStartFrame" {
            n106 = Variant To Data(error in=w463, type=0 ("Current Frame"), Variant=w457) -> (data=w455:i32, error out=w460:errorcluster)
            n107 = Bundle By Name(cluster=w462, "Start Frame"=w455) -> (w461:T5)
          }
          frame "UpdateEndFrame" {
            n108 = Variant To Data(error in=w472, type=0 ("Current Frame"), Variant=w466) -> (data=w464:i32, error out=w469:errorcluster)
            n109 = Bundle By Name(cluster=w471, "End Frame"=w464) -> (w470:T5)
          }
          frame "SetPDCSetup" {
            w473 = cluster{"PDCLists":T8, "Value":T9} {"PDCLists"={"ResolutionList"=[], "RecordRateList"=[], "ShutterSpeedList"=[], "TriggerModeList"=[]}, "Value"={"Color Type"=enum."MONO", "Bit Depth"=0, "Resolution"=0, "Record Rate"=0, "Shutter Speed"=0, "Trigger Mode"=0, "Display"=enum."Live", "Auto Trigger"=FALSE}}  # PDCLoadedSetup
            n110 = Unbundle By Name(w474) -> ("PDCSettings.Simulate"=w483:bool, "DeviceNo"=w478:u32, "ChildNo"=w476:u32)
            n111 = Variant To Data(error in=w482, type=w473, Variant=w480) -> (data=w479:cluster{"PDCLists":T8, "Value":T9}, error out=w481:errorcluster)
            n112 = case shown="False" w483 {
              tunnel: w481 -> [w491 w517]
              tunnel: [w515 w517] -> w484
              tunnel: w479 -> [w511 _]
              tunnel: w478 -> [w490 _]
              tunnel: [w514 T5 {"DeviceNo"=0, "ChildNo"=1, "ColorType"=enum."MONO", "BitDepth"=0, "Resolution"={"Width"=0, "Height"=0}, "RecordRate"=0, "ShutterSpeed"=0, "TriggerMode"=0, "Display"=enum."LiveStop", "PDCRecordStatus"=enum."Live", "PlayFrames"=FALSE, "Start Frame"=0, "Current Frame"=0, "End Frame"=0, "RefImage8bit"=[], "RefImage16bit"=[], "Auto Trigger"=FALSE, "PDCSettings"={"Interface"=enum."Gigabit-Ethernet", "AutoSearch"=FALSE, "IP - AutoSearch"=[], "IP - Direct"=[], "Simulate"=FALSE}} ("PDCAllStates")] -> w477
              tunnel: w476 -> [w489 _]
              tunnel: w475 -> [w513 _]
              tunnel: w474 -> [w512 _]
              frame False {
                n113 = Unbundle By Name(w511) -> ("Value.Color Type"=w495:enum16{"MONO", "COLOR"}, "Value.Bit Depth"=w496:i8, "PDCLists.TriggerModeList"=w508:string[], "Value.Trigger Mode"=w503:u16, "PDCLists.ShutterSpeedList"=w509:string[], "Value.Shutter Speed"=w504:u16, "PDCLists.RecordRateList"=w510:string[], "Value.Record Rate"=w505:u16, "PDCLists.ResolutionList"=w507:string[], "Value.Resolution"=w506:u16)
                n114 = call "PDCConvertTrigg.vi"("TriggerValue"=w503, "TriggerStrings"=w508) -> ("TriggerMode"=w499:u32)  [unwired: 9 in]
                n115 = call "PDCConvertShutter.vi"("ShutterValue"=w504, "ShutterList"=w509) -> ("ShutterSpeed"=w501:u32)  [unwired: 9 in]
                n116 = call "PDCConvertRecRate.vi"("RecRateValue"=w505, "RecRateList"=w510) -> ("RecRate"=w502:u32)  [unwired: 9 in]
                n117 = call "PDCConvertResolution.vi"("ResValue"=w506, "ResStrings"=w507) -> ("Height"=w487:u32, "Width"=w488:u32)  [unwired: 8 in]
                n118 = call "PDC_SetResolutionROI.vi"("DeviceNo"=w490, "ChildNo"=w489, "Width"=w488, "Height"=w487, "error in (no error)"=w491) -> ("error out"=w492:errorcluster)  [unwired: 8 in, 2 out]
                n119 = call "PDC_SetRecordRate.vi"("error in (no error)"=w492, "Rate"=w502, "ChildNo"=w489, "DeviceNo"=w490) -> ("error out"=w500:errorcluster)  [unwired: 5 in, 2 out]
                n120 = call "PDC_SetShutterSpeedFps.vi"("error in (no error)"=w500, "Fps"=w501, "ChildNo"=w489, "DeviceNo"=w490) -> ("error out"=w498:errorcluster)  [unwired: 5 in, 2 out]
                n121 = call "PDC_SetTriggerMode.vi"("DeviceNo"=w490, "Mode"=w499, "error in (no error)"=w498) -> ("error out"=w497:errorcluster)  [unwired: 10 in, 2 out]
                n122 = call "PDC_SetBitDepth.vi"("error in (no error)"=w497, "Depth"=w496, "ChildNo"=w489, "DeviceNo"=w490) -> ("error out"=w494:errorcluster)  [unwired: 5 in, 2 out]
                n123 = call "PDC_SetColorType.vi"("error in (no error)"=w494, "Mode"=w495, "ChildNo"=w489, "DeviceNo"=w490) -> ("error out"=w493:errorcluster)  [unwired: 5 in, 2 out]
                n124 = call "PDCGetAndDisplay.vi"("error in (no error)"=w493, "PDCAllStates in"=w512, "DataDisplayQueue"=w513) -> ("error out"=w515:errorcluster, "PDCAllStates out"=w514:T5)  [unwired: 7 in]
              }
              frame True {
              }
            }
          }
          frame "SetStatus" {
            n125 = Unbundle By Name(w518) -> ("PDCSettings.Simulate"=w528:bool, "DeviceNo"=w522:u32, "ChildNo"=w520:u32)
            n126 = Variant To Data(error in=w527, type=PDCDisplay."Live" ("NewVal"), Variant=w525) -> (data=w524:T6, error out=w526:errorcluster)
            n127 = case shown="False" w528 {
              tunnel: w526 -> [w545 w569]
              tunnel: [w547 w569] -> w529
              tunnel: w524 -> [w538 _]
              tunnel: w522 -> [w540 _]
              tunnel: [w546 T5 {"DeviceNo"=0, "ChildNo"=1, "ColorType"=enum."MONO", "BitDepth"=0, "Resolution"={"Width"=0, "Height"=0}, "RecordRate"=0, "ShutterSpeed"=0, "TriggerMode"=0, "Display"=enum."LiveStop", "PDCRecordStatus"=enum."Live", "PlayFrames"=FALSE, "Start Frame"=0, "Current Frame"=0, "End Frame"=0, "RefImage8bit"=[], "RefImage16bit"=[], "Auto Trigger"=FALSE, "PDCSettings"={"Interface"=enum."Gigabit-Ethernet", "AutoSearch"=FALSE, "IP - AutoSearch"=[], "IP - Direct"=[], "Simulate"=FALSE}} ("PDCAllStates")] -> w521
              tunnel: w520 -> [w539 _]
              tunnel: w519 -> [w537 _]
              tunnel: w518 -> [w536 _]
              frame False {
                n128 = case shown="\"Live\", Default" w538 {
                  tunnel: w545 -> [w563 w565 w567]
                  tunnel: [w563 w565 w567] -> w544
                  tunnel: [w562 w564 w566] -> w543
                  frame "Live", Default {
                    w562 = u32 0  # STATUS_LIVE
                  }
                  frame "Memory" {
                    w564 = u32 1  # STATUS_PLAYBACK
                    # "Memory"
                  }
                  frame "LiveStop" {
                    w566 = u32 0  # STATUS_LIVE
                    # "Memory"
                  }
                }
                n129 = call "PDC_SetStatus.vi"("error in (no error)"=w544, "Mode"=w543, "DeviceNo"=w540) -> ("error out"=w542:errorcluster)  [unwired: 6 in, 2 out]
                n130 = case shown="\"Memory\"" w538 {
                  tunnel: w542 -> [w549 w561]
                  tunnel: [w549 w557] -> w541
                  tunnel: w540 -> [_ w560]
                  tunnel: w539 -> [_ w559]
                  tunnel: w537 -> [_ w556]
                  tunnel: [w548 w552] -> w535
                  tunnel: [w548 w551] -> w534
                  tunnel: [w548 w550] -> w533
                  frame Default {
                    w548 = 0 ("Start")
                  }
                  frame "Memory" {
                    n131 = call "PDC_GetMemFrameInfo.vi"("error in (no error)"=w561, "ChildNo"=w559, "DeviceNo"=w560) -> ("error out"=w558:errorcluster, "Frame"=w553:T10)  [unwired: 5 in, 2 out]
                    n132 = To Variant(anything=w553) -> (Variant=w555:variant)
                    n133 = call "EnqueueMessage.vi"("error in (no error)"=w558, "MessageData"=w555, "Message"="DisplayMemFrameInfo", "MessageQueue"=w556) -> ("error out"=w557:errorcluster)  [unwired: 6 in, 1 out]
                    n134 = Unbundle By Name(w553) -> ("Start"=w552:i32, "End"=w551:i32, "Trigger"=w550:i32)
                  }
                }
                n135 = Bundle By Name(cluster=w536, "Start Frame"=w535, "End Frame"=w534, "Current Frame"=w533) -> (w532:T5)
                n136 = call "PDCGetAndDisplay.vi"("error in (no error)"=w541, "PDCAllStates in"=w532, "DataDisplayQueue"=w537) -> ("error out"=w547:errorcluster, "PDCAllStates out"=w546:T5)  [unwired: 7 in]
              }
              frame True {
              }
            }
          }
          frame "SetColorType" {
            n137 = Unbundle By Name(w570) -> ("PDCSettings.Simulate"=w580:bool, "DeviceNo"=w575:u32, "ChildNo"=w573:u32)
            n138 = Variant To Data(error in=w579, type=enum16{"MONO", "COLOR"}."MONO" ("ColorType"), Variant=w577) -> (data=w576:enum16{"MONO", "COLOR"}, error out=w578:errorcluster)
            n139 = case shown="False" w580 {
              tunnel: w578 -> [w588 w594]
              tunnel: [w592 w594] -> w581
              tunnel: w576 -> [w587 _]
              tunnel: w575 -> [w585 _]
              tunnel: [w591 T5 {"DeviceNo"=0, "ChildNo"=1, "ColorType"=enum."MONO", "BitDepth"=0, "Resolution"={"Width"=0, "Height"=0}, "RecordRate"=0, "ShutterSpeed"=0, "TriggerMode"=0, "Display"=enum."LiveStop", "PDCRecordStatus"=enum."Live", "PlayFrames"=FALSE, "Start Frame"=0, "Current Frame"=0, "End Frame"=0, "RefImage8bit"=[], "RefImage16bit"=[], "Auto Trigger"=FALSE, "PDCSettings"={"Interface"=enum."Gigabit-Ethernet", "AutoSearch"=FALSE, "IP - AutoSearch"=[], "IP - Direct"=[], "Simulate"=FALSE}} ("PDCAllStates")] -> w574
              tunnel: w573 -> [w586 _]
              tunnel: w572 -> [w590 _]
              tunnel: w570 -> [w584 _]
              frame False {
                n140 = call "PDC_SetColorType.vi"("error in (no error)"=w588, "Mode"=w587, "ChildNo"=w586, "DeviceNo"=w585) -> ("error out"=w589:errorcluster)  [unwired: 5 in, 2 out]
                n141 = call "PDCGetAndDisplay.vi"("error in (no error)"=w589, "PDCAllStates in"=w584, "DataDisplayQueue"=w590) -> ("error out"=w592:errorcluster, "PDCAllStates out"=w591:T5)  [unwired: 7 in]
              }
              frame True {
              }
            }
          }
          frame "SetBitDepth" {
            n142 = Variant To Data(error in=w604, type=i8 0 ("NewVal"), Variant=w602) -> (data=w601:i8, error out=w603:errorcluster)
            n143 = Unbundle By Name(w595) -> ("PDCSettings.Simulate"=w605:bool, "DeviceNo"=w600:u32, "ChildNo"=w598:u32)
            n144 = case shown="False" w605 {
              tunnel: w603 -> [w614 w619]
              tunnel: [w617 w619] -> w606
              tunnel: w601 -> [w613 _]
              tunnel: w600 -> [w611 _]
              tunnel: [w610 T5 {"DeviceNo"=0, "ChildNo"=1, "ColorType"=enum."MONO", "BitDepth"=0, "Resolution"={"Width"=0, "Height"=0}, "RecordRate"=0, "ShutterSpeed"=0, "TriggerMode"=0, "Display"=enum."LiveStop", "PDCRecordStatus"=enum."Live", "PlayFrames"=FALSE, "Start Frame"=0, "Current Frame"=0, "End Frame"=0, "RefImage8bit"=[], "RefImage16bit"=[], "Auto Trigger"=FALSE, "PDCSettings"={"Interface"=enum."Gigabit-Ethernet", "AutoSearch"=FALSE, "IP - AutoSearch"=[], "IP - Direct"=[], "Simulate"=FALSE}} ("PDCAllStates")] -> w599
              tunnel: w598 -> [w612 _]
              tunnel: w597 -> [w616 _]
              tunnel: w595 -> [w609 _]
              frame False {
                n145 = call "PDC_SetBitDepth.vi"("error in (no error)"=w614, "Depth"=w613, "ChildNo"=w612, "DeviceNo"=w611) -> ("error out"=w615:errorcluster)  [unwired: 5 in, 2 out]
                n146 = call "PDCGetAndDisplay.vi"("error in (no error)"=w615, "PDCAllStates in"=w609, "DataDisplayQueue"=w616) -> ("error out"=w617:errorcluster, "PDCAllStates out"=w610:T5)  [unwired: 7 in]
              }
              frame True {
              }
            }
          }
          frame "SetResolution" {
            w621 = cluster{"Width":u32, "Height":u32} {"Width"=0, "Height"=0}  # Resolution
            n147 = Variant To Data(error in=w629, type=w621, Variant=w627) -> (data=w622:cluster{"Width":u32, "Height":u32}, error out=w628:errorcluster)
            n148 = Unbundle By Name(w620) -> ("PDCSettings.Simulate"=w630:bool, "DeviceNo"=w626:u32, "ChildNo"=w624:u32)
            n149 = case shown="False" w630 {
              tunnel: w628 -> [w641 w646]
              tunnel: [w644 w646] -> w631
              tunnel: w626 -> [w640 _]
              tunnel: [w635 T5 {"DeviceNo"=0, "ChildNo"=1, "ColorType"=enum."MONO", "BitDepth"=0, "Resolution"={"Width"=0, "Height"=0}, "RecordRate"=0, "ShutterSpeed"=0, "TriggerMode"=0, "Display"=enum."LiveStop", "PDCRecordStatus"=enum."Live", "PlayFrames"=FALSE, "Start Frame"=0, "Current Frame"=0, "End Frame"=0, "RefImage8bit"=[], "RefImage16bit"=[], "Auto Trigger"=FALSE, "PDCSettings"={"Interface"=enum."Gigabit-Ethernet", "AutoSearch"=FALSE, "IP - AutoSearch"=[], "IP - Direct"=[], "Simulate"=FALSE}} ("PDCAllStates")] -> w625
              tunnel: w624 -> [w639 _]
              tunnel: w623 -> [w643 _]
              tunnel: w622 -> [w638 _]
              tunnel: w620 -> [w634 _]
              frame False {
                n150 = Unbundle By Name(w638) -> ("Width"=w636:u32, "Height"=w637:u32)
                n151 = call "PDC_SetResolution.vi"("DeviceNo"=w640, "ChildNo"=w639, "Width"=w636, "Height"=w637, "error in (no error)"=w641) -> ("error out"=w642:errorcluster)  [unwired: 8 in, 2 out]
                n152 = call "PDCGetAndDisplay.vi"("error in (no error)"=w642, "PDCAllStates in"=w634, "DataDisplayQueue"=w643) -> ("error out"=w644:errorcluster, "PDCAllStates out"=w635:T5)  [unwired: 7 in]
              }
              frame True {
              }
            }
          }
          frame "SetRecordRate" {
            n153 = Variant To Data(error in=w656, type=u32 0 ("number"), Variant=w654) -> (data=w653:u32, error out=w655:errorcluster)
            n154 = Unbundle By Name(w647) -> ("PDCSettings.Simulate"=w657:bool, "DeviceNo"=w652:u32, "ChildNo"=w650:u32)
            n155 = case shown="False" w657 {
              tunnel: w655 -> [w666 w671]
              tunnel: [w669 w671] -> w658
              tunnel: w653 -> [w665 _]
              tunnel: w652 -> [w664 _]
              tunnel: [w662 T5 {"DeviceNo"=0, "ChildNo"=1, "ColorType"=enum."MONO", "BitDepth"=0, "Resolution"={"Width"=0, "Height"=0}, "RecordRate"=0, "ShutterSpeed"=0, "TriggerMode"=0, "Display"=enum."LiveStop", "PDCRecordStatus"=enum."Live", "PlayFrames"=FALSE, "Start Frame"=0, "Current Frame"=0, "End Frame"=0, "RefImage8bit"=[], "RefImage16bit"=[], "Auto Trigger"=FALSE, "PDCSettings"={"Interface"=enum."Gigabit-Ethernet", "AutoSearch"=FALSE, "IP - AutoSearch"=[], "IP - Direct"=[], "Simulate"=FALSE}} ("PDCAllStates")] -> w651
              tunnel: w650 -> [w663 _]
              tunnel: w649 -> [w668 _]
              tunnel: w647 -> [w661 _]
              frame False {
                n156 = call "PDC_SetRecordRate.vi"("error in (no error)"=w666, "Rate"=w665, "ChildNo"=w663, "DeviceNo"=w664) -> ("error out"=w667:errorcluster)  [unwired: 5 in, 2 out]
                n157 = call "PDCGetAndDisplay.vi"("error in (no error)"=w667, "PDCAllStates in"=w661, "DataDisplayQueue"=w668) -> ("error out"=w669:errorcluster, "PDCAllStates out"=w662:T5)  [unwired: 7 in]
              }
              frame True {
              }
            }
          }
          frame "SetShutterSpeed" {
            n158 = Variant To Data(error in=w681, type=u32 0 ("number"), Variant=w679) -> (data=w678:u32, error out=w680:errorcluster)
            n159 = Unbundle By Name(w672) -> ("PDCSettings.Simulate"=w682:bool, "DeviceNo"=w677:u32, "ChildNo"=w675:u32)
            n160 = case shown="False" w682 {
              tunnel: w680 -> [w691 w696]
              tunnel: [w694 w696] -> w683
              tunnel: w678 -> [w688 _]
              tunnel: w677 -> [w690 _]
              tunnel: [w687 T5 {"DeviceNo"=0, "ChildNo"=1, "ColorType"=enum."MONO", "BitDepth"=0, "Resolution"={"Width"=0, "Height"=0}, "RecordRate"=0, "ShutterSpeed"=0, "TriggerMode"=0, "Display"=enum."LiveStop", "PDCRecordStatus"=enum."Live", "PlayFrames"=FALSE, "Start Frame"=0, "Current Frame"=0, "End Frame"=0, "RefImage8bit"=[], "RefImage16bit"=[], "Auto Trigger"=FALSE, "PDCSettings"={"Interface"=enum."Gigabit-Ethernet", "AutoSearch"=FALSE, "IP - AutoSearch"=[], "IP - Direct"=[], "Simulate"=FALSE}} ("PDCAllStates")] -> w676
              tunnel: w675 -> [w689 _]
              tunnel: w674 -> [w693 _]
              tunnel: w672 -> [w686 _]
              frame False {
                n161 = call "PDC_SetShutterSpeedFps.vi"("error in (no error)"=w691, "Fps"=w688, "ChildNo"=w689, "DeviceNo"=w690) -> ("error out"=w692:errorcluster)  [unwired: 5 in, 2 out]
                n162 = call "PDCGetAndDisplay.vi"("error in (no error)"=w692, "PDCAllStates in"=w686, "DataDisplayQueue"=w693) -> ("error out"=w694:errorcluster, "PDCAllStates out"=w687:T5)  [unwired: 7 in]
              }
              frame True {
              }
            }
          }
          frame "SetTriggerMode" {
            n163 = Variant To Data(error in=w706, type=u32 0 ("number"), Variant=w704) -> (data=w703:u32, error out=w705:errorcluster)
            n164 = Unbundle By Name(w697) -> ("PDCSettings.Simulate"=w707:bool, "DeviceNo"=w702:u32, "ChildNo"=w700:u32)
            n165 = case shown="False" w707 {
              tunnel: w705 -> [w715 w720]
              tunnel: [w718 w720] -> w708
              tunnel: w703 -> [w713 _]
              tunnel: w702 -> [w714 _]
              tunnel: [w712 T5 {"DeviceNo"=0, "ChildNo"=1, "ColorType"=enum."MONO", "BitDepth"=0, "Resolution"={"Width"=0, "Height"=0}, "RecordRate"=0, "ShutterSpeed"=0, "TriggerMode"=0, "Display"=enum."LiveStop", "PDCRecordStatus"=enum."Live", "PlayFrames"=FALSE, "Start Frame"=0, "Current Frame"=0, "End Frame"=0, "RefImage8bit"=[], "RefImage16bit"=[], "Auto Trigger"=FALSE, "PDCSettings"={"Interface"=enum."Gigabit-Ethernet", "AutoSearch"=FALSE, "IP - AutoSearch"=[], "IP - Direct"=[], "Simulate"=FALSE}} ("PDCAllStates")] -> w701
              tunnel: w700 -> [_ _]
              tunnel: w699 -> [w717 _]
              tunnel: w697 -> [w711 _]
              frame False {
                n166 = call "PDC_SetTriggerMode.vi"("DeviceNo"=w714, "Mode"=w713, "error in (no error)"=w715) -> ("error out"=w716:errorcluster)  [unwired: 10 in, 2 out]
                n167 = call "PDCGetAndDisplay.vi"("error in (no error)"=w716, "PDCAllStates in"=w711, "DataDisplayQueue"=w717) -> ("error out"=w718:errorcluster, "PDCAllStates out"=w712:T5)  [unwired: 7 in]
              }
              frame True {
              }
            }
          }
          frame "StartLogging" {
          }
          frame "StopLogging" {
          }
          frame "Stop" {
            n168 = Unbundle By Name(w731) -> ("PDCSettings.Simulate"=w730:bool, "DeviceNo"=w729:u32)
            n169 = case shown="False" w730 {
              tunnel: w733 -> [w738 w739]
              tunnel: [w737 w739] -> w732
              tunnel: w729 -> [w736 _]
              frame False {
                n170 = call "PDC_CloseDevice.vi"("error in (no error)"=w738, "DeviceNo"=w736) -> ("error out"=w737:errorcluster)  [unwired: 7 in, 2 out]
              }
              frame True {
              }
            }
          }
          frame "PDCPause" {
            n171 = Flush Queue(queue=w742, error in (no error)=w741) -> (error out=w740:errorcluster)  [unwired: 2 out]
            n172 = Unbundle By Name(w746) -> ("PDCSettings.Simulate"=w745:bool, "DeviceNo"=w744:u32)
            n173 = case shown="False" w745 {
              tunnel: w740 -> [w751 w752]
              tunnel: [w750 w752] -> w747
              tunnel: w744 -> [w749 _]
              frame False {
                n174 = call "PDC_CloseDevice.vi"("error in (no error)"=w751, "DeviceNo"=w749) -> ("error out"=w750:errorcluster)  [unwired: 7 in, 2 out]
              }
              frame True {
              }
            }
          }
        }
        n175 = call "ErrorModule.vi"("Error In"=w19, "CommunicationRefs"=w18) -> ("Error Out"=w20:errorcluster)  [unwired: 9 in]
      }
    }
    frame Error {
    }
  }
  "Error Out" <- w2
